vi "OhmsNumberToStringWithUnit.vi"(7 "ADC OVERRANGE":bool, 9 "ADC READING":dbl format="%#_13g", 11 "RANGE":i16(ring)=3 items=["2 MOhms"=7, "200 kOhms"=6, "20 kOhms"=5, "2 kOhms"=4, "200 Ohms"=3, "20 Ohms"=2, "2 Ohms"=1, "NO RANGE"=0]) -> (2 "RESISTANCE STRING":string="000.000 ohm")   [LabVIEW 2012]
doc: "Converts ADC reading+range info to\na string with unit (ohms, kohms Mohms)\nfor informative viewing on screen display"
panel:
  # "OhmsNumberToStringWithUnit.vi"
  # "RV-ELEKTRONIIKKA OY\nPICOWATT"
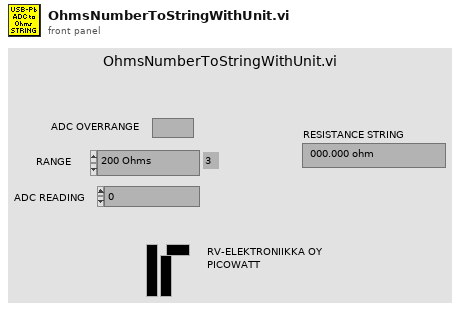
[diagram p1: front panel]
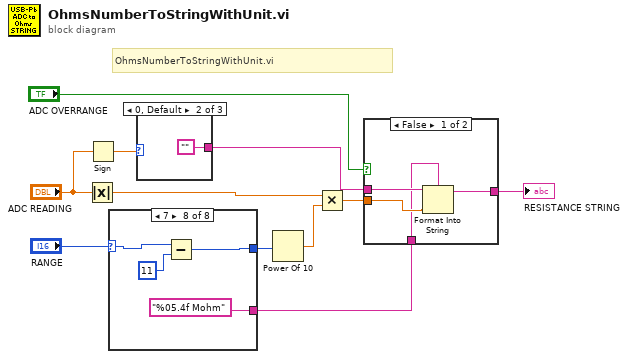
[diagram p0: block diagram]
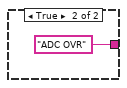
[diagram p2: hidden frame]
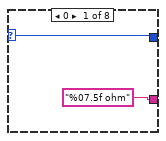
[diagram p3: hidden frame]
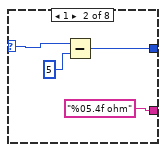
[diagram p4: hidden frame]
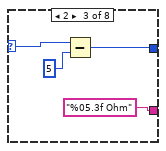
[diagram p5: hidden frame]
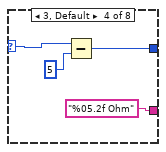
[diagram p6: hidden frame]
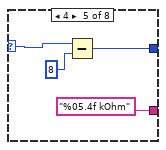
[diagram p7: hidden frame]
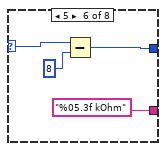
[diagram p8: hidden frame]
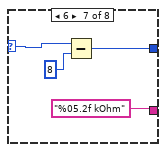
[diagram p9: hidden frame]
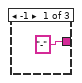
[diagram p10: hidden frame]
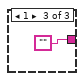
[diagram p11: hidden frame]
diagram:
  # "OhmsNumberToStringWithUnit.vi"
  n1 = Absolute Value(x="ADC READING") -> (abs(x)=w4:dbl)
  n2 = Sign(1:"ADC READING") -> (0:w8:dbl)
  n3 = case shown="7" "RANGE" {
    selector: "RANGE" -> [w12 w15 w20 w23 w26 w30 w35 w39]
    tunnel: ["%07.5f ohm" "%05.4f ohm" ("format string") "%05.3f Ohm" ("format string") "%05.2f Ohm" ("format string") "%05.4f kOhm" ("format string") "%05.3f kOhm" ("format string") "%05.2f kOhm" ("format string") "%05.4f Mohm" ("format string")] -> w6
    tunnel: [w12 w14 w18 w22 w27 w31 w34 w38] -> w1
    frame 0 {
    }
    frame 1 {
      n4 = Subtract(x=w15, y=u8 5) -> (x-y=w14:i16)
    }
    frame 2 {
      n5 = Subtract(x=w20, y=u8 5) -> (x-y=w18:i16)
    }
    frame 3, Default {
      n6 = Subtract(x=w23, y=u8 5) -> (x-y=w22:i16)
    }
    frame 4 {
      n7 = Subtract(x=w26, y=u8 8) -> (x-y=w27:i16)
    }
    frame 5 {
      n8 = Subtract(x=w30, y=u8 8) -> (x-y=w31:i16)
    }
    frame 6 {
      n9 = Subtract(x=w35, y=u8 8) -> (x-y=w34:i16)
    }
    frame 7 {
      n10 = Subtract(x=w39, y=u8 11) -> (x-y=w38:i16)
    }
  }
  n11 = case shown="0, Default" w8 {
    tunnel: ["-" "" ""] -> w7
    frame -1 {
    }
    frame 0, Default {
    }
    frame 1 {
    }
  }
  n12 = Power Of 10(x=w1) -> (10^x=w5:dbl)
  n13 = Multiply(x=w4, y=w5) -> (x*y=w9:dbl)
  n14 = case shown="False" "ADC OVERRANGE" {
    tunnel: [w48 "ADC OVR"] -> w10
    tunnel: w9 -> [w47 _]
    tunnel: w7 -> [w46 _]
    tunnel: w6 -> [w45 _]
    frame False {
      n15 = Format Into String(format string=w45, initial string=w46, w47) -> (resulting string=w48:string)  [unwired: 1 in, 1 out]
    }
    frame True {
    }
  }
  "RESISTANCE STRING" <- w10
